vi "设定三角形顶点.vi"(7 "端点C":T1 caption="点", 8 "error in (no error)":errorcluster caption="错误输入（无错误）", 9 "端点B":T1 caption="点", 10 "端点A":T1 caption="点", 11 "三角形 输入":refnum<class "三角形.lvclass"> caption="DNL_LabVIEW Object in") -> (0 "error out":errorcluster caption="错误输出", 3 "三角形 输出":refnum<class "三角形.lvclass"> caption="DNL_LabVIEW Object out")   [LabVIEW 2011, in "三角形.lvclass"]
uses:
  <vilib>/Utility/miscctls.llb/LVPointDoubleTypeDef.ctl
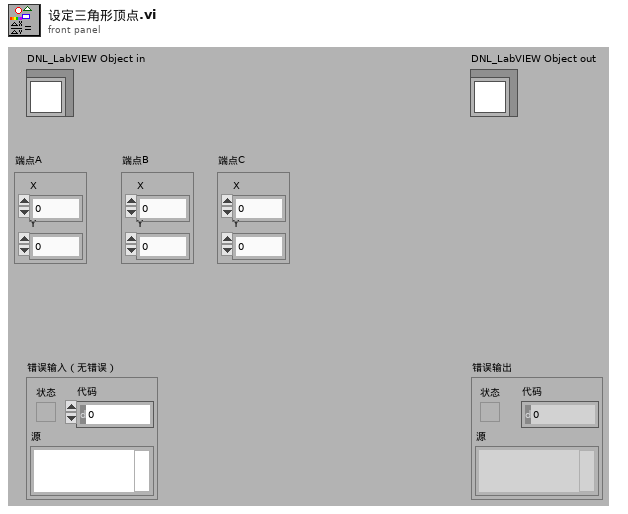
[diagram p1: front panel]
types:
  T1 = typedef "LVPointDoubleTypeDef.ctl" = cluster{"X":dbl, "Y":dbl}
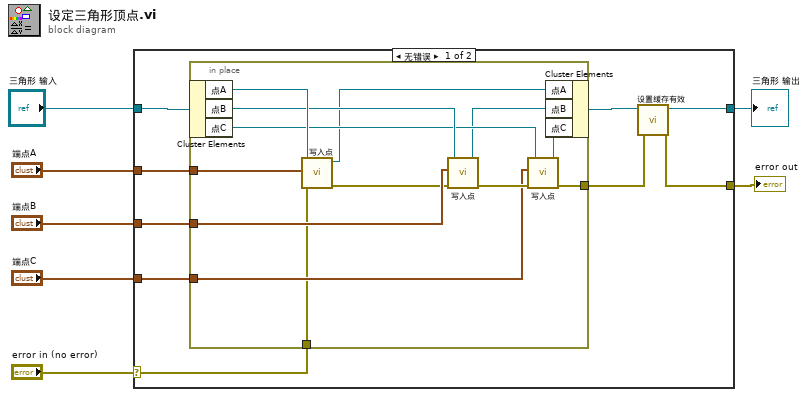
[diagram p0: block diagram]
diagram:
  n1 = case shown="无错误" "error in (no error)" {
    selector: "error in (no error)" -> [w10 w31]
    tunnel: [w8 w31] -> w6
    tunnel: [w11 w30] -> w4
    tunnel: "三角形 输入" -> [w16 w30]
    tunnel: "端点A" -> [w15 _]
    tunnel: "端点B" -> [w14 _]
    tunnel: "端点C" -> [w13 _]
    frame No Error {
      n2 = in-place {
        in-place-border: w15 -> [w29]
        in-place-border: w14 -> [w24]
        in-place-border: w13 -> [w23]
        in-place-border: w10 -> [w20]
        in-place-border: [w19] -> w9
        n3 = in-place-cluster #1(w16) -> ("点A"=w28:refnum<class "点.lvclass">, "点B"=w27:refnum<class "点.lvclass">, "点C"=w26:refnum<class "点.lvclass">)
        n4 = call "写入点.vi"("error in (no error)"=w20, "点"=w29, "点输入"=w28) -> ("error out"=w18:errorcluster, "点输出"=w17:refnum<class "点.lvclass">)  [unwired: 7 in]
        n5 = call "写入点.vi"("error in (no error)"=w18, "点"=w24, "点输入"=w27) -> ("error out"=w25:errorcluster, "点输出"=w22:refnum<class "点.lvclass">)  [unwired: 7 in]
        n6 = call "写入点.vi"("error in (no error)"=w25, "点"=w23, "点输入"=w26) -> ("error out"=w19:errorcluster, "点输出"=w21:refnum<class "点.lvclass">)  [unwired: 7 in]
        n7 = in-place-cluster #1("点A"=w17, "点B"=w22, "点C"=w21) -> (w12:refnum<class "三角形.lvclass">)
      }
      n8 = call "设置缓存有效.vi"("error in (no error)"=w9, "图形 输入"=w12) -> ("error out"=w8:errorcluster, "图形 输出"=w11:refnum<class "三角形.lvclass">)  [unwired: 8 in]
    }
    frame Error {
    }
  }
  "error out" <- w6
  "三角形 输出" <- w4
